vi "Immediate Initiate.vi"(8 "error in (no error)":errorcluster, 9 "Count Number (1)":i32=1, 10 "Channel (0: 1)":i32(ring) items=["1", "2", "Both"], 11 "VISA resource name":refnum<visa-resource-name>) -> (0 "error out":errorcluster, 3 "VISA resource name out":refnum<visa-resource-name>)   [LabVIEW 2019, in "Agilent 3352X Series.lvlib"]
doc: "Changes the triggering system from the OFF(\"idle\" state) to ON(the \"wait-for-trigger\" state) for specified number of triggers. \n\n<b>Note</b>:\nIf the triggering system is already turned ON by Continuous Initiate.VI, this vi will turn off the triggering system first then turn on it for specified trigger count."
uses:
  Agilent 3352X Series.lvlib
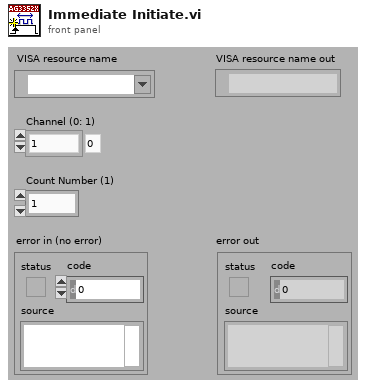
[diagram p1: front panel]
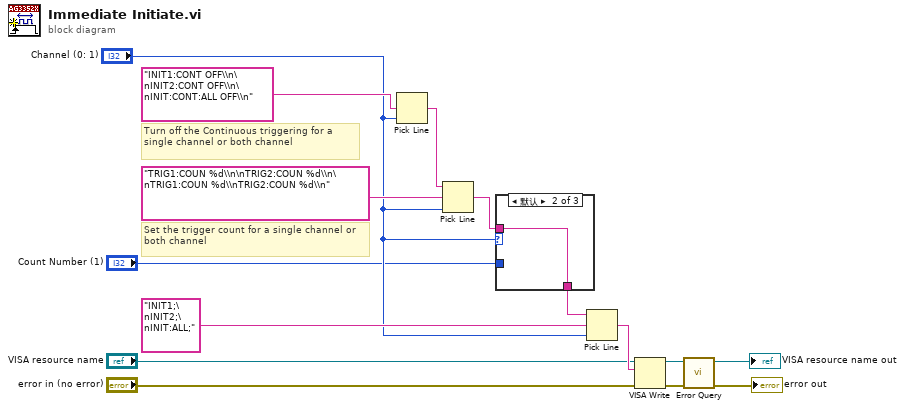
[diagram p0: block diagram]
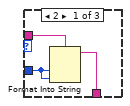
[diagram p2: hidden frame]
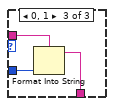
[diagram p3: hidden frame]
diagram:
  # "Set the trigger count for a single channel or both channel"
  # "Turn off the Continuous triggering for a single channel or both channel"
  n1 = Pick Line(multi-line string="INIT1:CONT OFF\\n\nINIT2:CONT OFF\\n\nINIT:CONT:ALL OFF\\n", line index="Channel (0: 1)") -> (output string=w12:string)  [unwired: 1 out]
  n2 = Pick Line(string ("")=w12, multi-line string="TRIG1:COUN %d\\n\nTRIG2:COUN %d\\n\nTRIG1:COUN %d\\nTRIG2:COUN %d\\n", line index="Channel (0: 1)") -> (output string=w9:string)
  n3 = case shown="默认" "Channel (0: 1)" {
    tunnel: [w17 w19 w22] -> w11
    tunnel: w9 -> [w18 w19 w21]
    tunnel: "Count Number (1)" -> [w16 _ w20]
    frame 2 {
      n4 = Format Into String(format string=w18, w16, w16) -> (resulting string=w17:string)  [unwired: 2 in, 1 out]
    }
    frame Default {
    }
    frame 0, 1 {
      n5 = Format Into String(format string=w21, w20) -> (resulting string=w22:string)  [unwired: 2 in, 1 out]
    }
  }
  n6 = Pick Line(string ("")=w11, multi-line string="INIT1;\nINIT2;\nINIT:ALL;", line index="Channel (0: 1)") -> (output string=w7:string)
  n7 = VISA Write(VISA resource name="VISA resource name", write buffer=w7, error in (no error)="error in (no error)") -> (VISA resource name out=w4:refnum<visa-resource-name>, error out=w3:errorcluster)  [unwired: 1 out]
  n8 = call "Error Query.vi"("error in (no error)"=w3, "VISA resource name"=w4) -> ("error out"=→"error out":errorcluster, "VISA resource name out"=→"VISA resource name out":refnum<visa-resource-name>)  [unwired: 8 out]
